vi "List.vi"(8 "error in (no error)":errorcluster) -> (0 "error out":errorcluster, 3 "registered loggers":string[](array[string]))   [LabVIEW 2024, in "Logging.lvlib" / "Registry.lvlib"]
uses:
  Registry.lvlib
  Registry Actions.ctl
  Utilities/Utilities.lvlib
panel:
  # "Connector Pane"
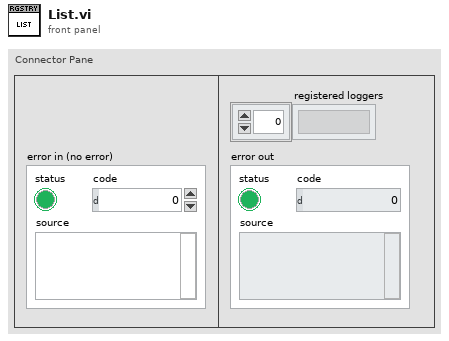
[diagram p1: front panel]
types:
  T1 = typedef "Logging.lvlib/Registry.lvlib/Registry Actions.ctl" = enum16{"Register", "Log", "List", "Unregister", "Unregister All"}
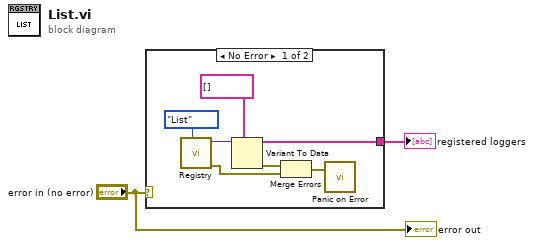
[diagram p0: block diagram]
diagram:
  n1 = case shown="No Error" "error in (no error)" {
    tunnel: [w6 _] -> w2
    frame No Error {
      n2 = call "Registry.vi"("action"=Registry_Actions."List") -> ("error out"=w4:errorcluster, "data out"=w8:variant)  [unwired: 9 in]
      n3 = Variant To Data(type=string[] [], Variant=w8) -> (data=w6:string[], error out=w5:errorcluster)  [unwired: 1 in]
      n4 = Merge Errors(w5, w4) -> (w3:errorcluster)
      n5 = call "Panic on Error.vi"("error in (no error)"=w3) -> ()  [unwired: 3 in]
    }
    frame Error {
    }
  }
  "registered loggers" <- w2
  "error out" <- "error in (no error)"
